vi "Process Snap Data.vi"(5 "Trigger Source":string, 6 "Timeout":bool, 7 "Polarity selector":u16, 8 "error in (no error)":errorcluster, 11 "Waveform Data":waveform(dbl)[](array[waveform])) -> (0 "error out":errorcluster, 1 "Pulse Width":dbl, 2 "Slope":dbl, 3 "Waveform Data out":waveform(dbl)[](array[waveform]))   [LabVIEW 2019, in "AnalogInput.lvlib" / "AnalogInput.lvclass"]
uses:
  Library/AnalogInput.lvclass
  <vilib>/measure/mascope.llb/Transition Measurements 1 chan.vi
  <vilib>/measure/NI_MAPro.lvlib
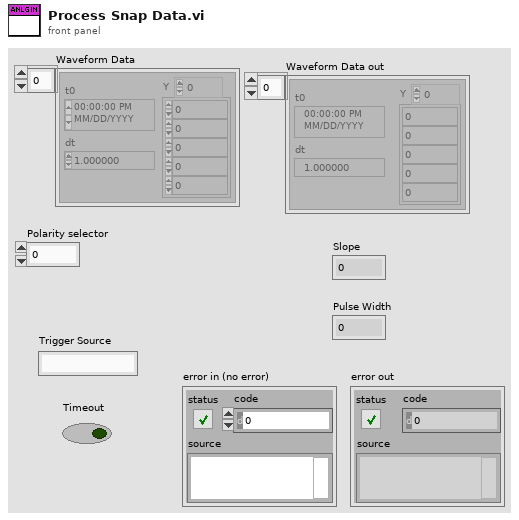
[diagram p1: front panel]
types:
  T1 = cluster{"high ref level":dbl, "mid ref level":dbl, "low ref level":dbl, "ref units":u16}
  T2 = cluster{"start time":dbl, "end time":dbl, "ref levels":cluster{"high ref level":dbl, "mid ref level":dbl, "low ref level":dbl, "ref units":u16}}
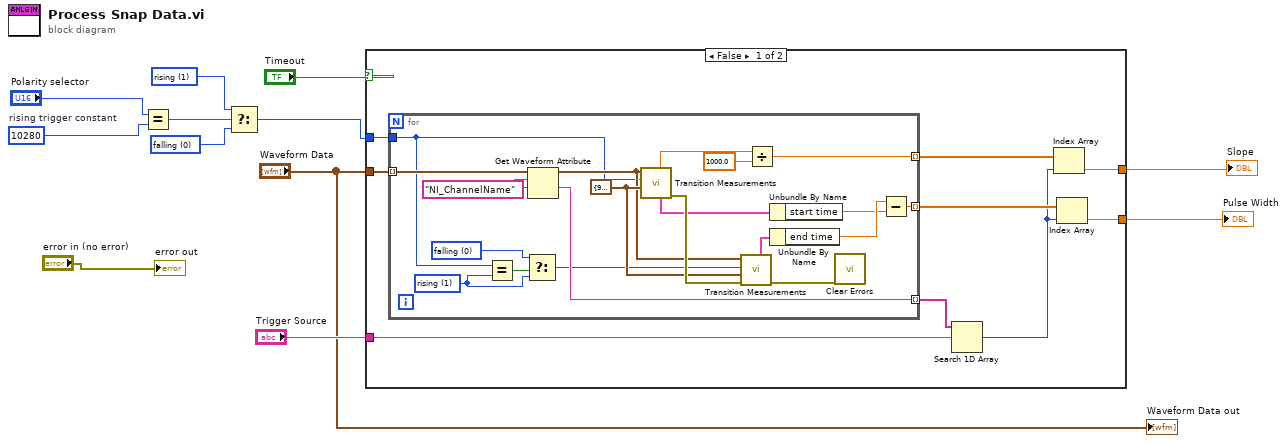
[diagram p0: block diagram]
diagram:
  w10 = u16 0 items=["falling", "rising"] ("polarity (rising)")
  w9 = u16 1 items=["falling", "rising"] ("polarity (rising)")
  w6 = 10280  # rising trigger constant
  n1 = Equal?(x="Polarity selector", y=w6) -> (x = y?=w8:bool)
  n2 = Select(t=w9, s=w8, f=w10) -> (s? t:f=w11:u16)
  n3 = case shown="False" "Timeout" {
    tunnel: "Waveform Data" -> [w21 _]
    tunnel: w11 -> [w20 _]
    tunnel: "Trigger Source" -> [w19 _]
    tunnel: [w16 _] -> w3
    tunnel: [w13 _] -> w5
    frame False {
      n4 = for {
        tunnel: w21 -> [w37] mode=indexing
        tunnel: w20 -> [w27]
        tunnel: [w39] -> w17 mode=indexing
        tunnel: [w36] -> w18 mode=indexing
        tunnel: [w28] -> w15 mode=indexing
        w24 = u16 0 items=["falling", "rising"] ("polarity (rising)")
        w25 = u16 1 items=["falling", "rising"] ("polarity (rising)")
        w38 = "NI_ChannelName" ("name")
        w34 = T1 {"high ref level"=90.0, "mid ref level"=50.0, "low ref level"=10.0, "ref units"=1} ("reference levels")
        n5 = Equal?(x=w27, y=w25) -> (x = y?=w26:bool)
        n6 = Select(t=w24, s=w26, f=w25) -> (s? t:f=w23:u16)
        n7 = Get Waveform Attribute(5:w38, 6:w38, 7:w37) -> (1:w36:string, 3:w32:waveform(dbl))  [unwired: 1 in, 2 out]
        n8 = call-poly <vilib>:"Transition Measurements.vi"("reference levels"=w34, "polarity (rising)"=w27, "signal in"=w32) -> ("error out"=w35:errorcluster, "measurement info"=w33:T2, "slope"=w41:dbl)  [unwired: 3 in, 3 out]
        n9 = call-poly <vilib>:"Transition Measurements.vi"("error in (no error)"=w35, "reference levels"=w34, "polarity (rising)"=w23, "signal in"=w32) -> ("error out"=w22:errorcluster, "measurement info"=w31:T2)  [unwired: 2 in, 4 out]
        n10 = Divide(x=w41, y=1000.0) -> (x/y=w39:dbl)
        n11 = Unbundle By Name(w33) -> ("start time"=w29:dbl)
        n12 = Unbundle By Name(w31) -> ("end time"=w30:dbl)
        n13 = call <vilib>:"Clear Errors.vi"("error in (no error)"=w22) -> ()  [unwired: 5 in, 2 out]
        n14 = Subtract(x=w30, y=w29) -> (x-y=w28:dbl)
      }
      n15 = Search 1D Array(1D array=w18, element=w19) -> (index of element=w14:i32)  [unwired: 1 in]
      n16 = Index Array(array=w17, index=w14) -> (element=w16:dbl)
      n17 = Index Array(array=w15, index=w14) -> (element=w13:dbl)
    }
    frame True {
    }
  }
  "Slope" <- w3
  "Pulse Width" <- w5
  "Waveform Data out" <- "Waveform Data"
  "error out" <- "error in (no error)"
